vi "SetClassQueue.vi"(8 "ErrorIn(No Error)":errorcluster caption="entrée d'erreur (pas d'erreur)", 11 "BaseDevice.lvclass":refnum<class "BaseDevice.lvclass">) -> (0 "sortie d'erreur":errorcluster, 3 "BaseDevice.lvclass Out":refnum<class "BaseDevice.lvclass">)   [LabVIEW 2010, in "BaseDevice.lvclass"]
uses:
  BaseDevice.lvclass
  BaseDevice.lvclass/BaseDevice.ctl
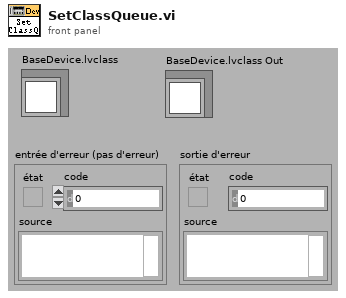
[diagram p1: front panel]
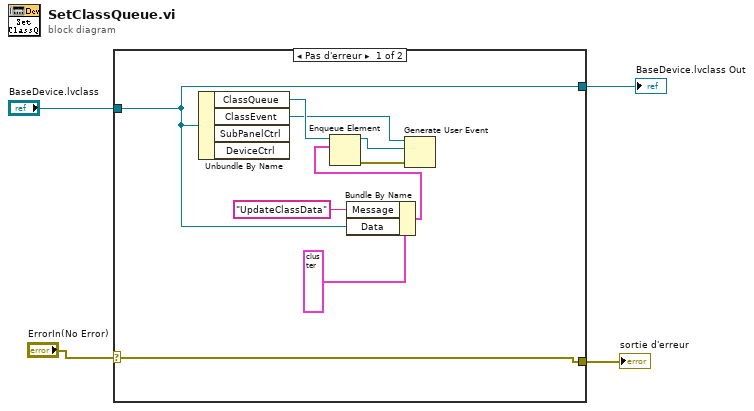
[diagram p0: block diagram]
diagram:
  n1 = case shown="Pas d'erreur" "ErrorIn(No Error)" {
    selector: "ErrorIn(No Error)" -> [w6 w15]
    tunnel: [w6 w15] -> w4
    tunnel: "BaseDevice.lvclass" -> [w5 w14]
    tunnel: [w5 w14] -> w1
    frame No Error {
      n2 = Unbundle By Name(w5) -> ("ClassQueue"=w11:refnum<queue>, "ClassEvent"=w10:refnum<user-event>)  [unwired: 2 out]
      n3 = Bundle By Name(cluster=cluster{"Message":string, "Data":variant, i32} {"Message"="", "Data"=variant, 0} ("élément"), "Message"="UpdateClassData", "Data"=w5) -> (w7:cluster{"Message":string, "Data":variant, i32})
      n4 = Enqueue Element(queue=w11, element=w7) -> (queue out=w13:refnum<queue>, error out=w12:errorcluster)  [unwired: 2 in, 1 out]
      n5 = Generate User Event(user event=w10, event data cluster=w13, error in=w12) -> ()  [unwired: 2 out]
    }
    frame Error {
    }
  }
  "sortie d'erreur" <- w4
  "BaseDevice.lvclass Out" <- w1
